vi "debug_glo.vi"() -> ()   [LabVIEW 2012]
panel:
  in  "random_line":dbl
  in  "chase":dbl
  in  "line":dbl
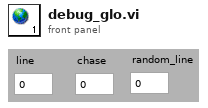
[diagram p1: front panel]
diagram:
